vi "Scope Base_Create.vi"(8 "Error In":errorcluster, 10 "IConfigure":refnum<class "IConfigure.lvclass">, 11 "reference in":refnum<class "Scope Base.lvclass">) -> (0 "Error Out":errorcluster, 3 "reference out":refnum<class "Scope Base.lvclass">)   [LabVIEW 2023, in "Scope Base.lvlib" / "Scope Base.lvclass"]
uses:
  Scope Base.lvclass
  Scope Base.lvclass/Scope Base.ctl
  Instrument Base/Instrument Base.lvclass
  D:/git/HAL/HAL GOOP4/Instrument Base/Instrument Base.lvclass
  D:/git/HAL/HAL GOOP4/Interfaces/IInstrument Base/IInstrument Base.lvclass
  D:/git/HAL/HAL GOOP4/Scope/Scope Base/Scope Base.lvclass
  Interfaces/IConfigure/IConfigure.lvclass
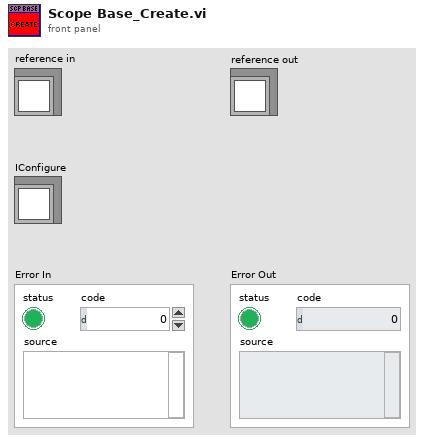
[diagram p1: front panel]
types:
  T1 = typedef "Scope Base.lvlib/Scope Base.lvclass/ObjectAttributes.ctl" = cluster{"Last Waveforms":map{u8, waveform(dbl)}}
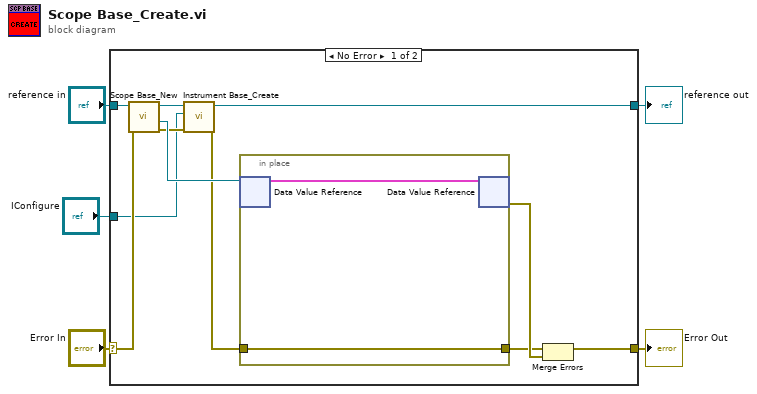
[diagram p0: block diagram]
diagram:
  n1 = case shown="No Error" "Error In" {
    selector: "Error In" -> [w12 w20]
    tunnel: [w10 w20] -> w4
    tunnel: "reference in" -> [w14 w19]
    tunnel: [w9 w19] -> w2
    tunnel: "IConfigure" -> [w6 _]
    frame No Error {
      n2 = call "Scope Base_New.vi"("Error In"=w12, "reference in"=w14) -> ("Error Out"=w13:errorcluster, "DVRRefOut"=w16:refnum<data-value>, "reference out"=w15:refnum<class "Scope Base.lvclass">)  [unwired: 6 in, 1 out]
      n3 = call "Instrument Base_Create.vi"("Error In"=w13, "IConfigure.lvclass"=w6, "reference in"=w15) -> ("Error Out"=w8:errorcluster, "reference out"=w9:refnum<class "Scope Base.lvclass">)  [unwired: 7 in]
      n4 = in-place {
        in-place-border: w8 -> [w18]
        in-place-border: [w18] -> w7
        n5 = in-place-dvr #1(w16) -> (w17:T1)  [unwired: 1 out]
        n6 = in-place-dvr #1(w17) -> (w11:errorcluster)  [unwired: 1 out]
      }
      n7 = Merge Errors(w7, w11) -> (w10:errorcluster)
    }
    frame Error {
    }
  }
  "Error Out" <- w4
  "reference out" <- w2
